vi "Test Joystic Sensitivity Youtube Arcade drive.vi"() -> ()   [LabVIEW 2017]
panel:
  in  "Z Angle":dbl
  out "Y Output":dbl
  out "X Output":dbl
  in  "x Input":dbl
  in  "y Input":dbl
  in  "n^x(Unbounded)":dbl=2.5 format="%#_13g"
  in  "Select Function":T1(ring)
  in  "Dead Zone(0 to 1)":dbl=0.01
  in  "Min Output(0 to 1)":dbl=0.1
  in  "Turn Rate":dbl=1.0
  in  "Speed Rate":dbl=1.0
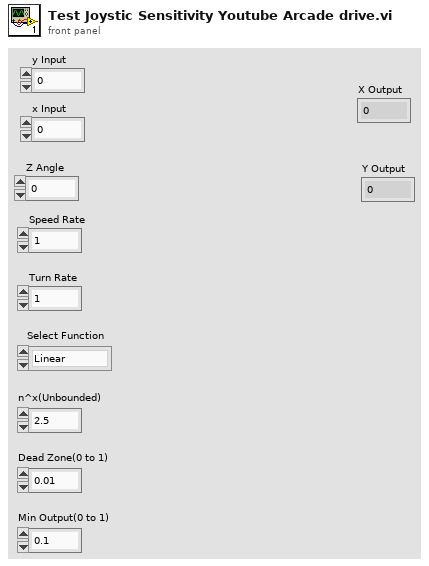
[diagram p1: front panel]
types:
  T1 = enum16{"Linear", "Square  Root", "Square", "n^x"}
  T2 = cluster{"X":dbl, "Y":dbl, "Angle":dbl, "Magnitude":dbl}
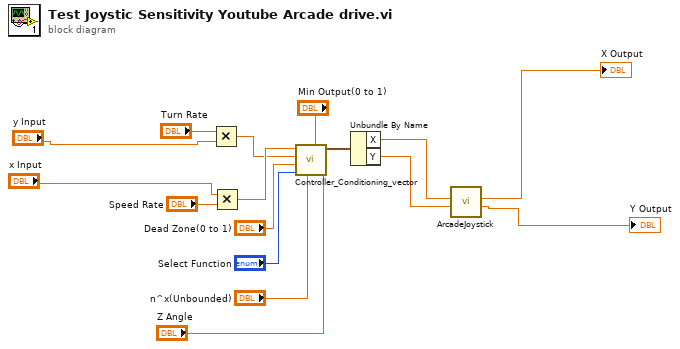
[diagram p0: block diagram]
diagram:
  n1 = Multiply(x="Turn Rate", y="y Input") -> (x*y=w13:dbl)
  n2 = Multiply(x="x Input", y="Speed Rate") -> (x*y=w14:dbl)
  n3 = call "Controller_Conditioning_vector.vi"("Angular Offset\n(-180 to 180 or 0 to 360)"="Z Angle", "Min Output(0 to 1)"="Min Output(0 to 1)", "n^x(Unbounded)"="n^x(Unbounded)", "Select Function"="Select Function", "Dead Zone(0 to 1)"="Dead Zone(0 to 1)", "Y(-1 to 1)"=w13, "X(-1 to 1)"=w14) -> ("output cluster"=w12:T2)  [unwired: 4 in]
  n4 = Unbundle By Name(w12) -> ("X"=w4:dbl, "Y"=w3:dbl)
  n5 = call "ArcadeJoystick.vi"("Y axis value"=w3, "X axis value"=w4) -> ("Right Motor Value"=→"Y Output":dbl, "Left Motor Value"=→"X Output":dbl)  [unwired: 8 in]
